vi "DC_init.vi"(8 "error in (no error)":errorcluster, 10 "Enable Motor(T)":bool=TRUE, 11 "KNR in":T1) -> (0 "error out":errorcluster, 3 "KNR out":T1, 4 "output\nposition 2":i32, 6 "output\nPosition_1":i32)   [LabVIEW 2013]
uses:
  <userlib>/KNR OS 3.0 LabVIEW Toolkit/Type Definition/KNR3 Reference.ctl
  <userlib>/_FPGA Interface Advanced Tools/FPGA Interface Base/FPGA Interface Base.lvclass
  <userlib>/KNR OS 3.0 LabVIEW Toolkit/Type Definition/Resource.ctl
  Global 1.vi
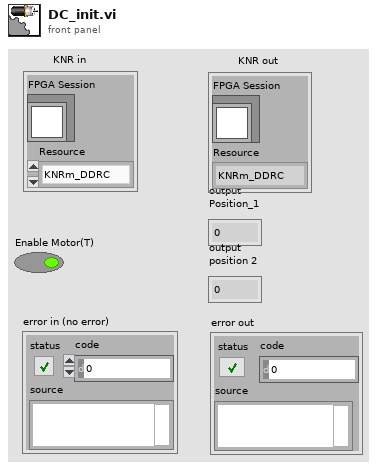
[diagram p1: front panel]
types:
  T1 = typedef "KNR3 Reference.ctl" = cluster{"FPGA Session":refnum<class "FPGA Interface Base.lvclass">, "Resource":T2}
  T2 = typedef "Resource.ctl" = enum16{"KNRm_DDRC", "KNRm_DDDD", "KNRm_DDDR", "KNRm_DDDC", "KNR"}
  T3 = typedef "DC Motor Port.ctl" = u16
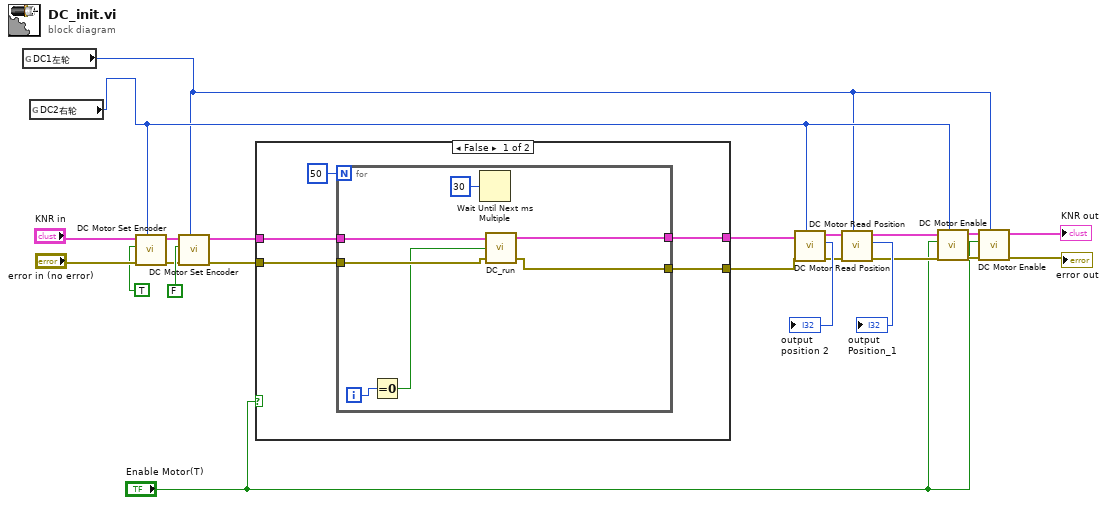
[diagram p0: block diagram]
diagram:
  n1 = global read "Global 1.vi" "DC1左轮"() -> (w1:T3)
  n2 = global read "Global 1.vi" "DC2右轮"() -> (w2:T3)
  n3 = call <userlib>:"DC Motor Set Encoder.vi"("Port (DS1)"=w2, "error in (no error)"="error in (no error)", "Reverse?(F)"=TRUE, "KNR in"="KNR in") -> ("error out"=w14:errorcluster, "KNR out"=w15:T1)  [unwired: 6 in]
  n4 = call <userlib>:"DC Motor Set Encoder.vi"("Port (DS1)"=w1, "error in (no error)"=w14, "Reverse?(F)"=FALSE ("5V Power"), "KNR in"=w15) -> ("error out"=w5:errorcluster, "KNR out"=w6:T1)  [unwired: 6 in]
  n5 = case shown="False" "Enable Motor(T)" {
    tunnel: w6 -> [w25 w36]
    tunnel: w5 -> [w27 w37]
    tunnel: [w24 w36] -> w4
    tunnel: [w26 w37] -> w3
    frame False {
      n6 = for {
        N: 50 -> [_]
        tunnel: w27 -> [w34]
        tunnel: [w31] -> w26
        tunnel: w25 -> [w30]
        tunnel: [w29] -> w24
        i -> [w33]
        n7 = Equal To 0?(x=w33) -> (x = 0?=w32:bool)
        n8 = Wait Until Next ms Multiple(millisecond multiple=u32 30) -> ()  [unwired: 1 out]
        n9 = call "DC_run.vi"("KNR in"=w30, "reinitialize? (F)"=w32, "error in (no error)"=w34) -> ("KNR out"=w29:T1, "error out"=w31:errorcluster)  [unwired: 3 in, 2 out]
      }
    }
    frame True {
    }
  }
  n10 = call <userlib>:"DC Motor Read Position.vi"("Port (DS1)"=w2, "error in (no error)"=w3, "KNR in"=w4) -> ("error out"=w21:errorcluster, "Position"=→"output\nposition 2":i32, "KNR out"=w20:T1)  [unwired: 6 in]
  n11 = call <userlib>:"DC Motor Read Position.vi"("Port (DS1)"=w1, "error in (no error)"=w21, "KNR in"=w20) -> ("error out"=w8:errorcluster, "Position"=→"output\nPosition_1":i32, "KNR out"=w9:T1)  [unwired: 6 in]
  n12 = call <userlib>:"DC Motor Enable.vi"("Port (DS1)"=w2, "error in (no error)"=w8, "Enable Motor(F)"="Enable Motor(T)", "KNR in"=w9) -> ("error out"=w12:errorcluster, "KNR out"=w13:T1)  [unwired: 6 in]
  n13 = call <userlib>:"DC Motor Enable.vi"("Port (DS1)"=w1, "error in (no error)"=w12, "Enable Motor(F)"="Enable Motor(T)", "KNR in"=w13) -> ("error out"=→"error out":errorcluster, "KNR out"=→"KNR out":T1)  [unwired: 6 in]
